vi "IPI_Cal_Step1_Left.vi"(8 "error in":errorcluster, 10 "Image In":T1, 11 "Session In":T2) -> (0 "error out":errorcluster, 2 "mm":sgl, 3 "Image":T1(plugin-control), 4 "x = 0?":bool)   [LabVIEW 2015]
uses:
  <vilib>/userdefined/High Color/IMAQdx.ctl
  <vilib>/vision/Image Controls.llb/IMAQ Image.ctl
  <vilib>/vision/Measure.llb/Edge Options.ctl
  <vilib>/vision/Measure.llb/Edge Polarity.ctl
  <vilib>/vision/driver/NI_Vision_Acquisition_Software.lvlib
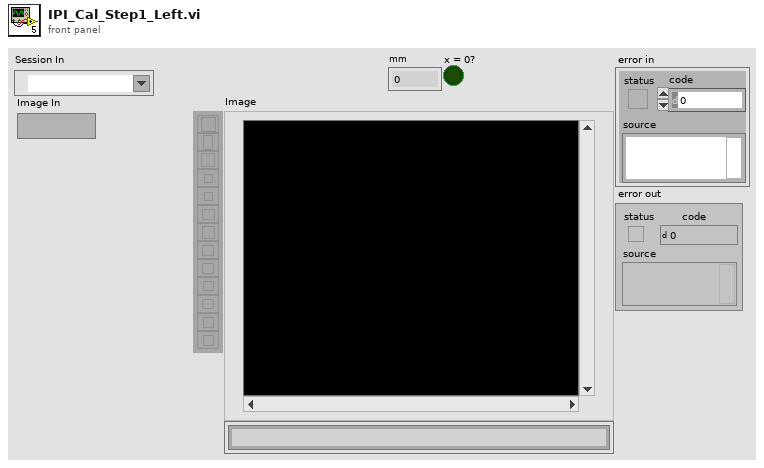
[diagram p1: front panel]
types:
  T1 = typedef "IMAQ Image.ctl" = refnum<image>
  T2 = typedef "IMAQdx.ctl" = refnum<k21>
  T3 = typedef "Edge Options.ctl" = cluster{"Edge Polarity":T4, "Kernel Size":u32, "Width":u32, "Minimum Edge Strength":sgl, "Interpolation Type":enum32{"Zero Order", "Bilinear", "Quadratic", "Cubic", "Bilinear Fixed"}, "Data Processing Method":enum32{"Average", "Median"}}
  T4 = typedef "Edge Polarity.ctl" = u32
  T5 = cluster{"Search Direction":u32, "Edge Options":T3, "Show Search Area":bool, "Show Search Lines":bool, "Show Edges Found":bool, "Show Result":bool, "Search Area Color":u32, "Search Lines Color":u32, "Edge Locations Color":u32, "Result Color":u32, "Overlay Group Name":string}
  T6 = cluster{"Global Rectangle":i32[], "Contours":cluster{"ID":enum32{"External", "Internal"}, "Type":u32, "Coordinates":i32[]}[]}
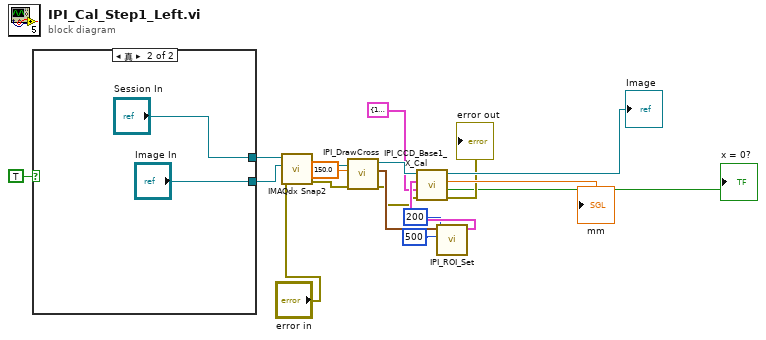
[diagram p0: block diagram]
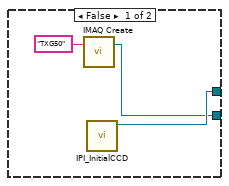
[diagram p2: hidden frame]
diagram:
  n1 = case shown="真" TRUE {
    tunnel: [w21 "Session In"] -> w10
    tunnel: [w19 "Image In"] -> w9
    frame False {
      n2 = call "IMAQ Create"("Image Name"="TXG50") -> ("New Image"=w19:T1)  [unwired: 4 in, 1 out]
      n3 = call "IPI_InitialCCD.vi"() -> ("Session Out"=w21:T2)  [unwired: 10 in, 1 out]
    }
    frame True {
    }
  }
  n4 = call <vilib>:"IMAQdx Snap2.vi"("error in"="error in", "Image In"=w9, "Session In"=w10) -> ("error out"=w6:errorcluster, "Image Out"=w18:T1)  [unwired: 6 in, 1 out]
  n5 = call "IPI_DrawCross.vi"("error in (no error)"=w6, "X"=150.0 ("R"), "Image In"=w18) -> ("error out"=w5:errorcluster, "XYCenter"=w15:cluster{"X":i32, "Y":i32}, "Image Out"=w16:T1)  [unwired: 6 in]
  n6 = call "IPI_ROI_Set.vi"("Y"=200 ("y"), "X"=500 ("R"), "XYCenter"=w15) -> ("ROI"=w13:T6)  [unwired: 8 in]
  n7 = call "IPI_CCD_Base1_X_Cal.vi"("error in"=w5, "Options (Find Straight Edge 1)"=T5 {"Search Direction"=1, "Edge Options"={"Edge Polarity"=0, "Kernel Size"=5, "Width"=1, "Minimum Edge Strength"=88.0, "Interpolation Type"=enum."Bilinear Fixed", "Data Processing Method"=enum."Average"}, "Show Search Area"=TRUE, "Show Search Lines"=TRUE, "Show Edges Found"=TRUE, "Show Result"=TRUE, "Search Area Color"=65280, "Search Lines Color"=255, "Edge Locations Color"=16776960, "Result Color"=16711680, "Overlay Group Name"=""}, "ROI Descriptor (Find Straight Edge 1)"=w13, "Image In"=w16) -> ("error out"=→"error out":errorcluster, "x = 0?"=→"x = 0?":bool, "mm"=→"mm":sgl, "Image"=→"Image":T1)  [unwired: 4 in]
